vi "Initialize Categories List.vi"(8 "error in (no error)":errorcluster, 11 "StoreUI in":refnum<class "StoreUI.lvclass">) -> (0 "error out":errorcluster, 2 "Icons":T1[](array[typedef]), 3 "StoreUI out":refnum<class "StoreUI.lvclass">)   [LabVIEW 2015, in "StoreUI.lvlib" / "StoreUI.lvclass"]
uses:
  StoreUI.lvclass
  <vilib>/picture/picture.llb/imagedata.ctl
  StoreUI.lvclass/StoreUI.ctl
  VI Store/VIStore Actor/VIStore.lvclass/VIStore.ctl
  Classes/Category/Category.lvclass
  VI Store/VIStore Actor/VIStore.lvclass
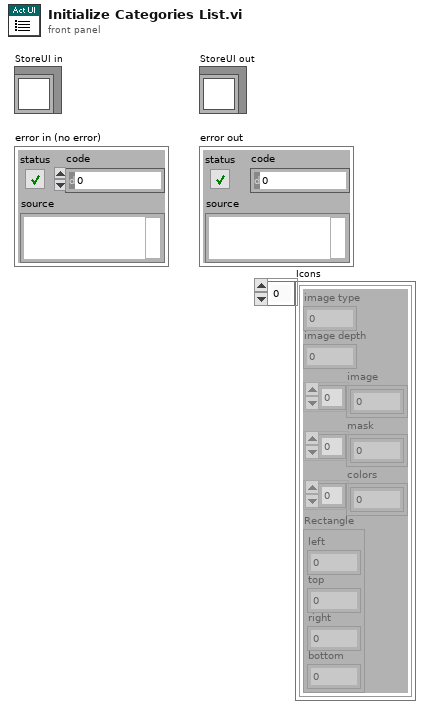
[diagram p1: front panel]
types:
  T1 = typedef "imagedata.ctl" = cluster{"image type":i32, "image depth":i32, "image":u8[], "mask":u8[], "colors":u32[], "Rectangle":cluster{"left":i16, "top":i16, "right":i16, "bottom":i16}}
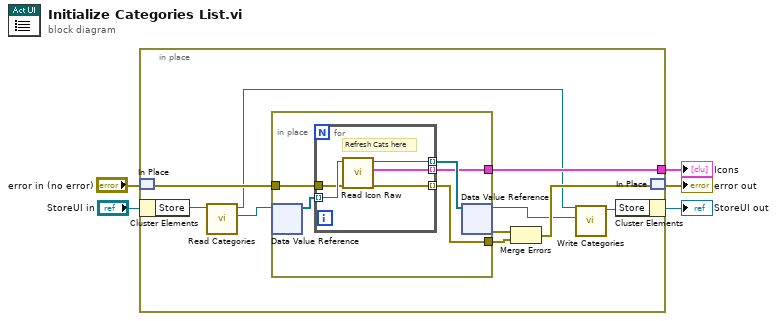
[diagram p0: block diagram]
diagram:
  n1 = in-place {
    in-place-border: [w11] -> w1
    n2 = in-place-match #1("error in (no error)") -> (w13:errorcluster)
    n3 = in-place-cluster #2("StoreUI in") -> ("Store"=w10:refnum<class "VIStore.lvclass">)
    n4 = call "Read Categories.vi"("VIStore in"=w10) -> ("Categories"=w9:refnum<data-value>, "VIStore out"=w6:refnum<class "VIStore.lvclass">)  [unwired: 8 in, 1 out]
    n5 = in-place {
      in-place-border: w13 -> [w17]
      in-place-border: [w18] -> w14
      in-place-border: [w16] -> w11
      n6 = in-place-dvr #3(w9) -> (w20:refnum<class "Category.lvclass">[])  [unwired: 1 out]
      n7 = for {
        tunnel: w20 -> [w25] mode=indexing
        tunnel: [w24] -> w19 mode=indexing
        tunnel: [w23] -> w16 mode=indexing
        tunnel: [w22] -> w18 mode=indexing
        tunnel: w17 -> [w21]
        # "Refresh Cats here"
        n8 = call-dynamic "Read Icon Raw.vi"("error in (no error)"=w21, "Category in"=w25) -> ("error out"=w22:errorcluster, "Icon Raw"=w23:T1, "Category out"=w24:refnum<class "Category.lvclass">)  [unwired: 7 in]
      }
      n9 = in-place-dvr #3(w19) -> (w8:refnum<data-value>, w15:errorcluster)
    }
    n10 = Merge Errors(w15, w14) -> (w12:errorcluster)
    n11 = call "Write Categories.vi"("Categories"=w8, "VIStore in"=w6) -> ("VIStore out"=w7:refnum<class "VIStore.lvclass">)  [unwired: 8 in, 1 out]
    n12 = in-place-cluster #2("Store"=w7) -> (→"StoreUI out":refnum<class "StoreUI.lvclass">)
    n13 = in-place-match #1(w12) -> (→"error out":errorcluster)
  }
  "Icons" <- w1
